vi "Power Spectrum Density.vi"(0 "Percentage":dbl, 4 "window parameter":dbl=nan, 5 "Data Valid":bool, 6 "averaging parameters":T1={"averaging mode"=enum."No averaging", "weighting mode"=enum."Exponential", "number of averages"=10} {"number of averages" min=1}, 7 "export mode":T3 items=["Power Spectrum", "Power Spectral Density"], 8 "dB":bool, 9 "window":T2=1 items=["Rectangle"=0, "Hanning"=1, "Hamming"=2, "Blackman-Harris"=3, "Exact Blackman"=4, "Blackman"=5, "Flat Top"=6, "4 Term B-Harris "=7, "7 Term B-Harris"=8, "Low Sidelobe"=9, "Blackman Nuttall"=11, "Triangle"=30, "Bartlett-Hanning"=31, "Bohman"=32, "Parzen"=33, "Welch"=34, "Kaiser"=60, "Dolph-Chebyshev"=61, "Gaussian"=62], 10 "Channel Name":string, 11 "Signal":waveform(dbl)={"t0"=timestamp(0 s since 1904-01-01), "dt"=0.0, "Y"=[]}) -> ()   [LabVIEW 2023, in "Power Spectrum Density.lvlib" / "Power Spectrum Density.lvclass"]
uses:
  Power Spectrum Density.lvclass
  <vilib>/measure/maspectr.llb/Power Spectrum and PSD Export Mode.ctl
  <vilib>/Analysis/4window.llb/windowTd.ctl
  <vilib>/measure/maspectr.llb/FFT Power Spectrum and PSD for 1 Chan.vi
  <vilib>/measure/NI_MAPro.lvlib
  <vilib>/Analysis/NI_AALPro.lvlib
panel:
  out "Buffering...":dbl(slide) scale=0.0..100.0
  in  "Restart averaging":bool
  out "Averages completed":dbl
  out "Power Spectrum":cluster{"f0":dbl, "df":dbl, "magnitude":dbl[]}(graph)
  out "Linear averaging done":bool
  out "Title":string
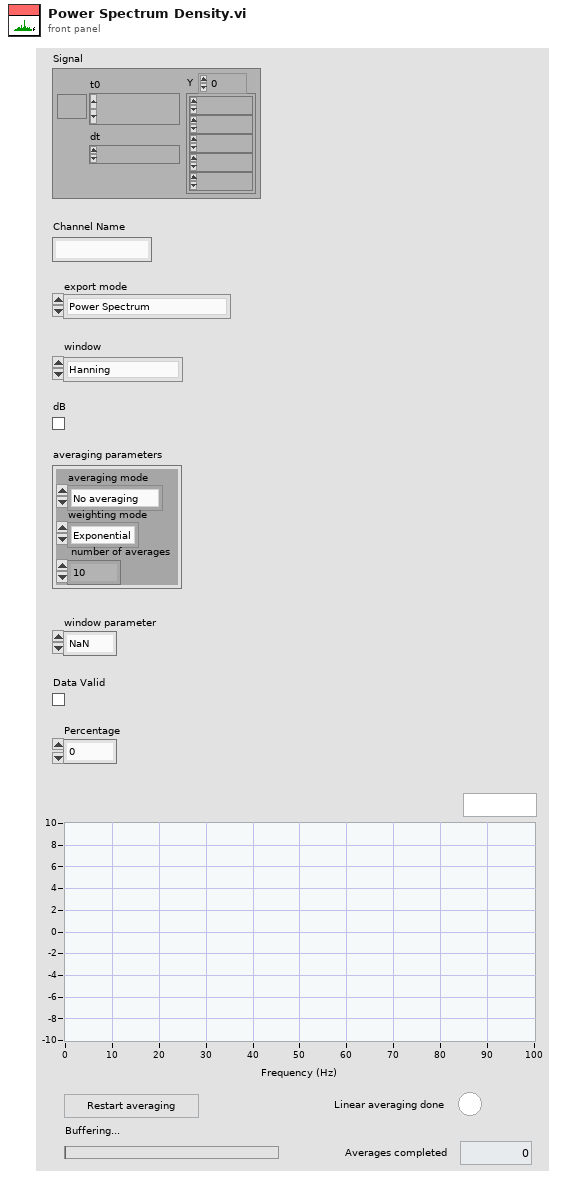
[diagram p1: front panel]
types:
  T1 = cluster{"averaging mode":enum16{"No averaging", "Vector averaging", "RMS averaging", "Peak hold"}, "weighting mode":enum16{"Linear", "Exponential"}, "number of averages":u32}
  T2 = typedef "NI_AALPro.lvlib/windowTd.ctl" = u32
  T3 = typedef "NI_MAPro.lvlib/Power Spectrum and PSD Export Mode.ctl" = u16
  T4 = cluster{"Power Spectrum / PSD":cluster{"f0":dbl, "df":dbl, "magnitude":dbl[]}, "averaging done":bool, "averages completed":dbl}
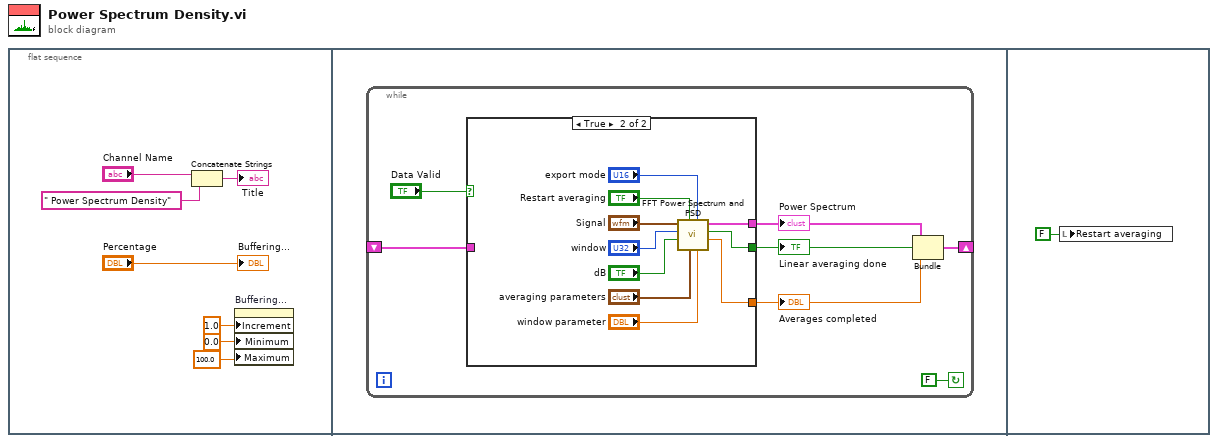
[diagram p0: block diagram]
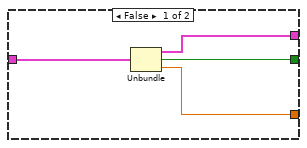
[diagram p2: hidden frame]
diagram:
  n1 = flat-sequence {
    frame #0 {
      n2 = Concatenate Strings("Channel Name", " Power Spectrum Density" ("string")) -> (→"Title":string)
      n3 = property on="Buffering..." class="Slide (strict)"("Increment"=1.0 ("Data Entry Limits:Increment"), "Minimum"=0.0 ("Data Entry Limits:Minimum"), "Maximum"=100.0 ("Data Entry Limits:Maximum")) -> ()  [unwired: 2 in, 2 out]
      "Buffering..." <- "Percentage"
    }
    frame #1 {
      n4 = while {
        shift-right: [w10] -> _
        shift-left: _ -> [w9]
        stop <- FALSE continue-if-true
        n5 = case shown="True" "Data Valid" {
          tunnel: [w17 w21] -> w11
          tunnel: [w15 w19] -> w12
          tunnel: [w18 w20] -> w13
          tunnel: w9 -> [w16 _]
          frame False {
            n6 = Unbundle(w16) -> ("Power Spectrum / PSD"=w18:cluster{"f0":dbl, "df":dbl, "magnitude":dbl[]}, "averaging done"=w15:bool, "averages completed"=w17:dbl)
          }
          frame True {
            n7 = call-poly <vilib>:"FFT Power Spectrum and PSD.vi"("window parameter"="window parameter", "export mode"="export mode", "averaging parameters"="averaging parameters", "restart averaging (F)"="Restart averaging", "dB On (F)"="dB", "window"="window", "time signal"="Signal") -> ("averages completed"=w21:dbl, "averaging done"=w19:bool, "Power Spectrum / PSD"=w20:cluster{"f0":dbl, "df":dbl, "magnitude":dbl[]})  [unwired: 1 in, 1 out]
          }
        }
        "Power Spectrum" <- w13
        "Linear averaging done" <- w12
        "Averages completed" <- w11
        n8 = Bundle("Power Spectrum / PSD"=w13, "averaging done"=w12, "averages completed"=w11) -> (w10:T4)  [unwired: 1 in]
      }
    }
    frame #2 {
      n9 = local write "Restart averaging"(FALSE ("Restart averaging")) -> ()
    }
  }
